vi "Lex.vi"   [LabVIEW 2018, in "Toolkit.lvlib"]
doc: "Reads a series of bytes and breaks it up into identified tokens. This is also known as \"tokenizing\", and it is the first action, or process, in compiling.\n\n<B>Input/Reader</B> - Either the Mustache template to tokenize or a reader capable of reading a Mustache template byte-by-byte. If the input is a string, a String reader will automatically be created.\n\n<B>Tokens</B> - The identified tokens from the Mustache template in order read order, i.e. element zero is the first identified token when reading the Mustache template from the beginning."
uses:
  Toolkit.lvlib
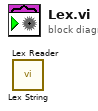
[diagram p0: block diagram]
diagram:
  n1 = call "Lex String.vi"() -> ()  [unwired: 10 in, 2 out]
  n2 = call "Lex Reader.vi"() -> ()  [unwired: 10 in, 2 out]
